vi "OphirRead.vi"(0 "OphirPM":T1, 11 "error in":errorcluster) -> (4 "Power (W)":dbl format="%.3p", 6 "Ophir Samples":i32, 15 "error out":errorcluster)   [LabVIEW 2012]
panel:
  # "OPHIR USBI Read"
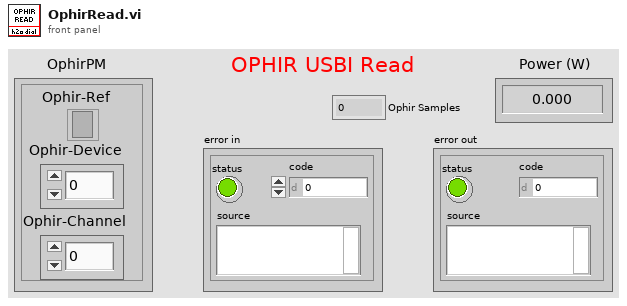
[diagram p1: front panel]
types:
  T1 = cluster{"Ophir-Ref":refnum<k7>, "Ophir-Device":i32, "Ophir-Channel":i32}
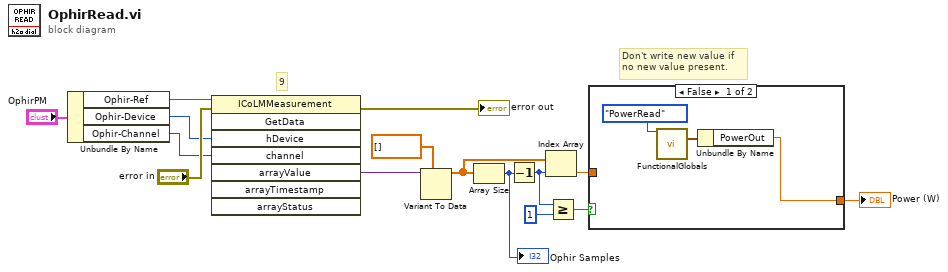
[diagram p0: block diagram]
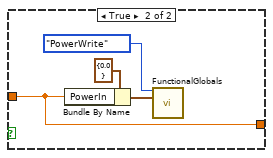
[diagram p2: hidden frame]
diagram:
  # "Don't write new value if\nno new value present."
  # "9"
  n1 = Unbundle By Name("OphirPM") -> ("Ophir-Ref"=w7:refnum<k7>, "Ophir-Device"=w6:i32, "Ophir-Channel"=w5:i32)
  n2 = invoke class="ICoLMMeasurement" method="GetData"(reference=w7, error in="error in", "hDevice"=w6, "channel"=w5) -> (error out=→"error out":errorcluster, "arrayValue"=w15:variant)  [unwired: 4 in, 6 out]
  n3 = Variant To Data(type=dbl[] [], Variant=w15) -> (data=w9:dbl[])  [unwired: 1 in, 1 out]
  n4 = Array Size(array=w9) -> (size(s)=w13:i32)
  "Ophir Samples" <- w13
  n5 = Decrement(x=w13) -> (x-1=w4:i32)
  n6 = Index Array(array=w9, index=w4) -> (element=w12:dbl)
  n7 = Greater Or Equal?(x=w4, y=1) -> (x >= y?=w2:bool)
  n8 = case shown="False" w2 {
    tunnel: w12 -> [_ w19]
    tunnel: [w16 w19] -> w1
    frame False {
      n9 = call "FunctionalGlobals.vi"("FG_Control"=enum16{"Initialize", "PowerRead", "PowerWrite"}."PowerRead") -> ("FG_OUT"=w17:cluster{"PowerOut":dbl})  [unwired: 14 in]
      n10 = Unbundle By Name(w17) -> ("PowerOut"=w16:dbl)
    }
    frame True {
      n11 = Bundle By Name(cluster=cluster{"PowerIn":dbl} {"PowerIn"=0.0} ("FG_IN"), "PowerIn"=w19) -> (w21:cluster{"PowerIn":dbl})
      n12 = call "FunctionalGlobals.vi"("FG_Control"=enum16{"Initialize", "PowerRead", "PowerWrite"}."PowerWrite", "FG_IN"=w21) -> ()  [unwired: 13 in, 1 out]
    }
  }
  "Power (W)" <- w1
